vi "Delete Generated Server Code.vi"(8 "error in (no error)":errorcluster, 11 "Project Path":path) -> (0 "error out":errorcluster)   [LabVIEW 2019, in "gRPC Template Creation Utility.lvlib"]
uses:
  gRPC Template Creation Utility.lvlib
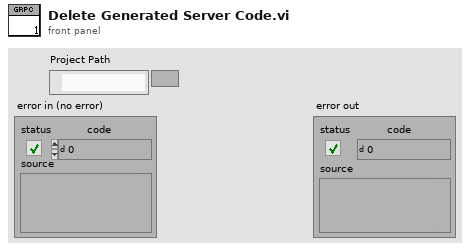
[diagram p1: front panel]
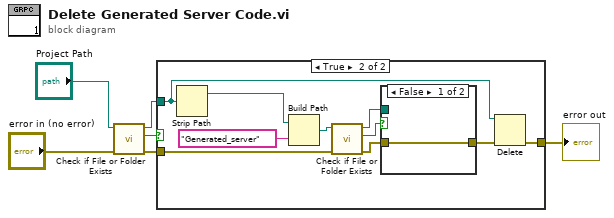
[diagram p0: block diagram]
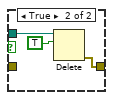
[diagram p3: hidden frame]
diagram:
  n1 = call <vilib>:"Check if File or Folder Exists.vi"("error in (no error)"="error in (no error)", "path"="Project Path") -> ("error out"=w3:errorcluster, "file or folder exists?"=w5:bool, "dup path"=w4:path)  [unwired: 7 in]
  n2 = case shown="True" w5 {
    tunnel: w4 -> [_ w11]
    tunnel: w3 -> [w7 w9]
    tunnel: [w7 w8] -> w1
    frame False {
    }
    frame True {
      n3 = Strip Path(path=w11) -> (stripped path=w10:path)  [unwired: 1 out]
      n4 = Build Path(base path=w10, name or relative path="Generated_server") -> (appended path=w16:path)
      n5 = call <vilib>:"Check if File or Folder Exists.vi"("error in (no error)"=w9, "path"=w16) -> ("error out"=w12:errorcluster, "file or folder exists?"=w14:bool, "dup path"=w15:path)  [unwired: 7 in]
      n6 = case shown="False" w14 {
        tunnel: w15 -> [_ w20]
        tunnel: [w18 w19] -> w13
        tunnel: w12 -> [w18 _]
        frame False {
        }
        frame True {
          n7 = Delete(path (use dialog)=w20, entire hierarchy (F)=TRUE) -> (error out=w19:errorcluster)  [unwired: 3 in, 2 out]
        }
      }
      n8 = Delete(path (use dialog)=w11, error in=w13) -> (error out=w8:errorcluster)  [unwired: 3 in, 2 out]
    }
  }
  "error out" <- w1
